vi "Unregister-user-events.vi"(8 "error in (no error)":errorcluster, 10 "Event Registration":refnum<event-registration>, 11 "ModComm in":T1) -> (0 "error out":errorcluster, 3 "ModComm out":T1)   [LabVIEW 2013, in "SLMServer.lvlib" / "SLMServer.lvclass"]
uses:
  SLMServer.lvclass
  Object-reference.ctl
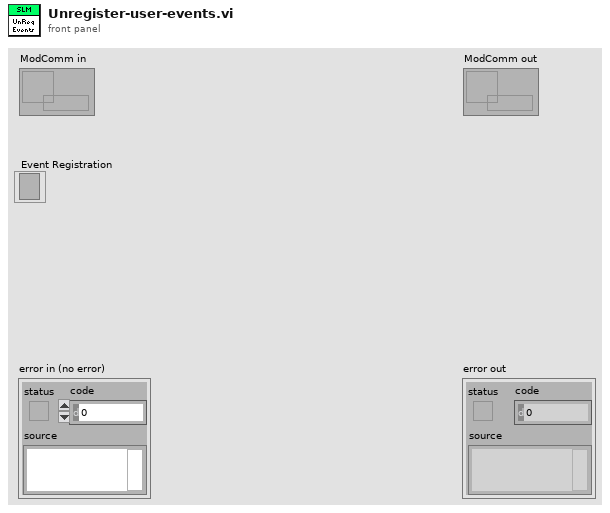
[diagram p1: front panel]
types:
  T1 = typedef "SLMServer.lvlib/SLMServer.lvclass/Object-reference.ctl" = refnum<data-value>
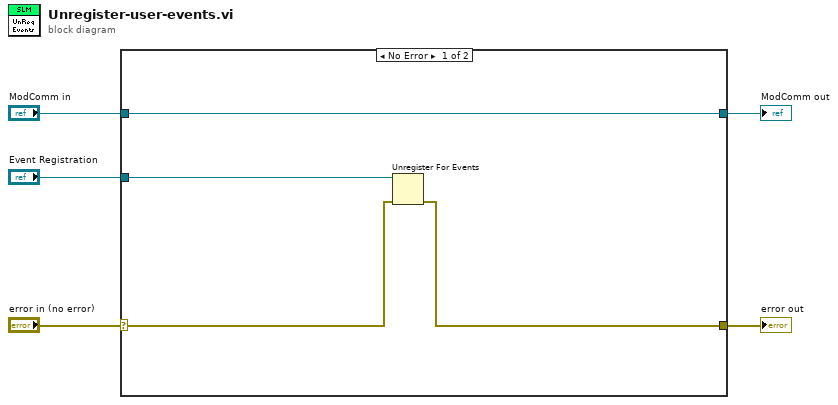
[diagram p0: block diagram]
diagram:
  n1 = case shown="No Error" "error in (no error)" {
    selector: "error in (no error)" -> [w8 w11]
    tunnel: [w6 w11] -> w4
    tunnel: [w9 w10] -> w2
    tunnel: "ModComm in" -> [w9 w10]
    tunnel: "Event Registration" -> [w7 _]
    frame No Error {
      n2 = Unregister For Events(event registration refnum=w7, error in=w8) -> (error out=w6:errorcluster)
    }
    frame Error {
    }
  }
  "error out" <- w4
  "ModComm out" <- w2
